vi "Add Recipe.vi"(8 "error in (no error)":errorcluster, 9 "Cluster":cluster{"Speed":u16, "Temp":u16, "Time":u16}, 11 "MASTER in":refnum<class "MASTER.lvclass">) -> (0 "error out":errorcluster, 3 "MASTER out":refnum<class "MASTER.lvclass">)   [LabVIEW 2014, in "Files Library.lvlib" / "MASTER.lvclass"]
uses:
  MASTER.lvclass
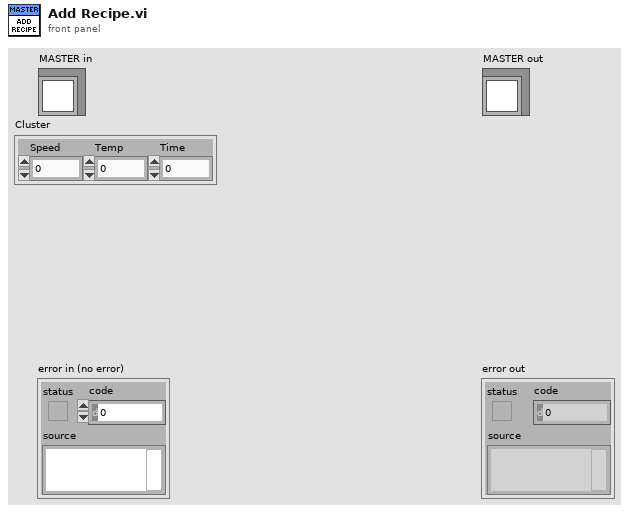
[diagram p1: front panel]
types:
  T1 = cluster{"Speed":u16, " Temperature Setpoint":u16, " Time Limit":u16}[]
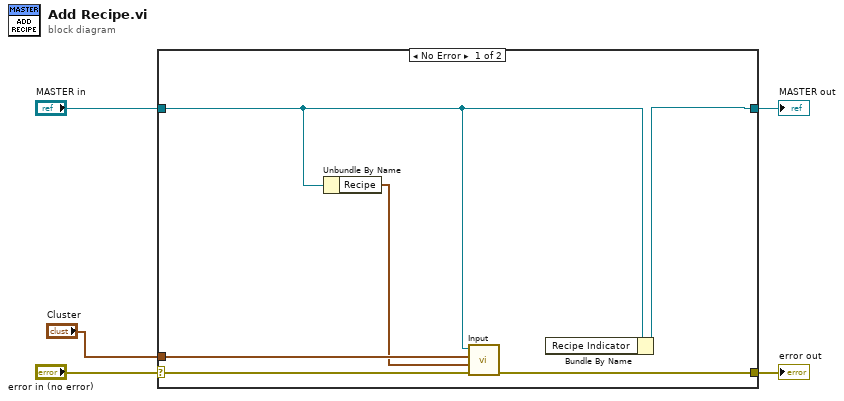
[diagram p0: block diagram]
diagram:
  n1 = case shown="No Error" "error in (no error)" {
    selector: "error in (no error)" -> [w11 w13]
    tunnel: [w10 w13] -> w4
    tunnel: [w7 w12] -> w2
    tunnel: "MASTER in" -> [w6 w12]
    tunnel: "Cluster" -> [w9 _]
    frame No Error {
      n2 = Unbundle By Name(w6) -> ("Recipe"=w8:T1)
      n3 = call-dynamic "Input.vi"("error in (no error)"=w11, "Dryer Control input"=w8, "Cluster"=w9, "MASTER in"=w6) -> ("error out"=w10:errorcluster)  [unwired: 6 in, 1 out]
      n4 = Bundle By Name(cluster=w6) -> (w7:refnum<class "MASTER.lvclass">)  [unwired: 1 in]
    }
    frame Error {
    }
  }
  "error out" <- w4
  "MASTER out" <- w2
